vi "SeimensS7Net_WriteInt16[].vi"(8 "error in (no error)":errorcluster caption="错误输入（无错误）", 9 "values":i16[](array[numeric]), 10 "address":string="DB600.0", 11 "Seimens 输入":refnum<class "Seimens.lvclass">) -> (0 "error out":errorcluster caption="错误输出", 2 "values 2":i16[](array[numeric]), 3 "Seimens 输出":refnum<class "Seimens.lvclass">)   [LabVIEW 2018, in "Seimens.lvclass"]
uses:
  Seimens.lvclass
  Seimens.lvclass/Seimens.ctl
  D:/LiMing/Labview/lib/LM_HslCommunication/DLL/HslCommunication.dll
  DLL/HslCommunication.dll
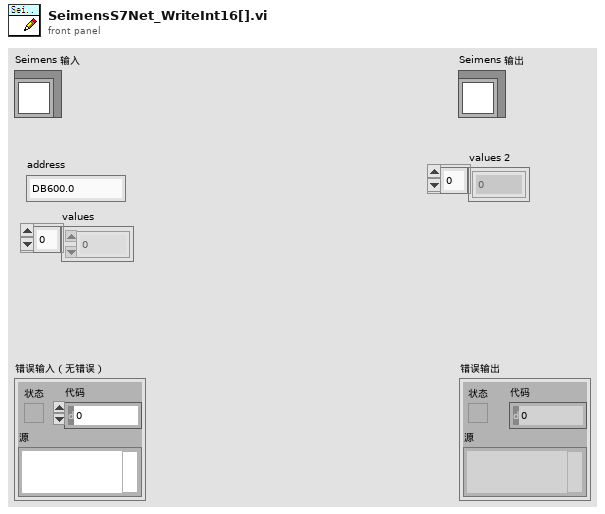
[diagram p1: front panel]
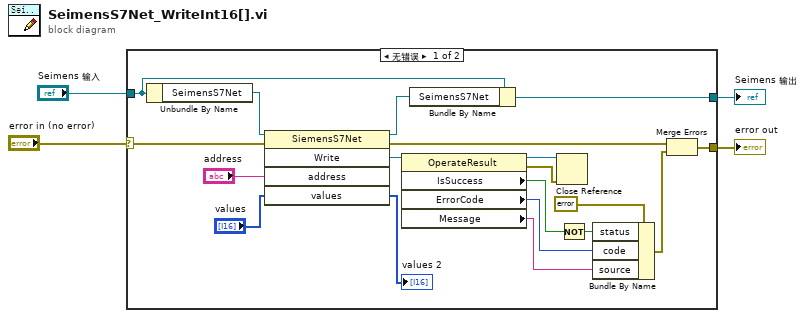
[diagram p0: block diagram]
diagram:
  n1 = case shown="无错误" "error in (no error)" {
    selector: "error in (no error)" -> [w9 w25]
    tunnel: [w8 w25] -> w3
    tunnel: [w11 w24] -> w1
    tunnel: "Seimens 输入" -> [w12 w24]
    frame No Error {
      n2 = Unbundle By Name(w12) -> ("SeimensS7Net"=w13:refnum<k24>)
      n3 = invoke class="SiemensS7Net" method="Write"(reference=w13, error in=w9, "address"="address", "values"="values") -> (reference out=w10:refnum<k24>, error out=w19:errorcluster, "Write"=w16:refnum<k24>, "values"=→"values 2":i16[])  [unwired: 1 in, 1 out]
      n4 = property class="OperateResult"(reference=w16) -> (reference out=w18:refnum<k24>, error out=w17:errorcluster, "IsSuccess"=w20:bool, "ErrorCode"=w21:i32, "Message"=w22:string)  [unwired: 1 in]
      n5 = Bundle By Name(cluster=w12, "SeimensS7Net"=w10) -> (w11:refnum<class "Seimens.lvclass">)
      n6 = Close Reference(reference=w18, error in (no error)=w17) -> ()  [unwired: 1 out]
      n7 = Not(x=w20) -> (.not. x?=w5:bool)
      n8 = Bundle By Name(cluster=errorcluster {"status"=FALSE, "code"=0, "source"=""} ("error in (no error)"), "status"=w5, "code"=w21, "source"=w22) -> (w23:errorcluster)
      n9 = Merge Errors(w19, w23) -> (w8:errorcluster)
    }
    frame Error {
    }
  }
  "error out" <- w3
  "Seimens 输出" <- w1
